vi "LEP_RV_InfoFile.vi"(0 "Path To Executable":path, 5 "Operation":u16(ring) items=["Read", "Write"], 7 "Item":string(combo), 9 "Data In":string, 11 "error in (no error)":errorcluster) -> (4 "Data Out":string, 15 "error out":errorcluster)   [LabVIEW 2011]
doc: "Loads project configuration information, creates the build folder, prepares the source files, builds, and links the embedded application."
uses:
  <vilib>/Utility/config.llb/Read Key (String).vi
  <vilib>/Utility/config.llb/Write Key (String).vi
  <vilib>/Utility/config.llb/NI_LVConfig.lvlib
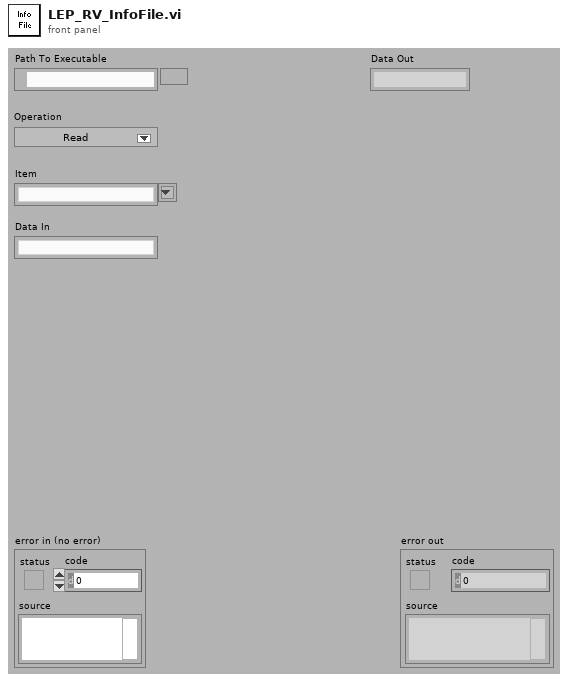
[diagram p1: front panel]
types:
  T1 = typedef "NI_LVConfig.lvlib/Config Data RefNum.ctl" = refnum<k1>
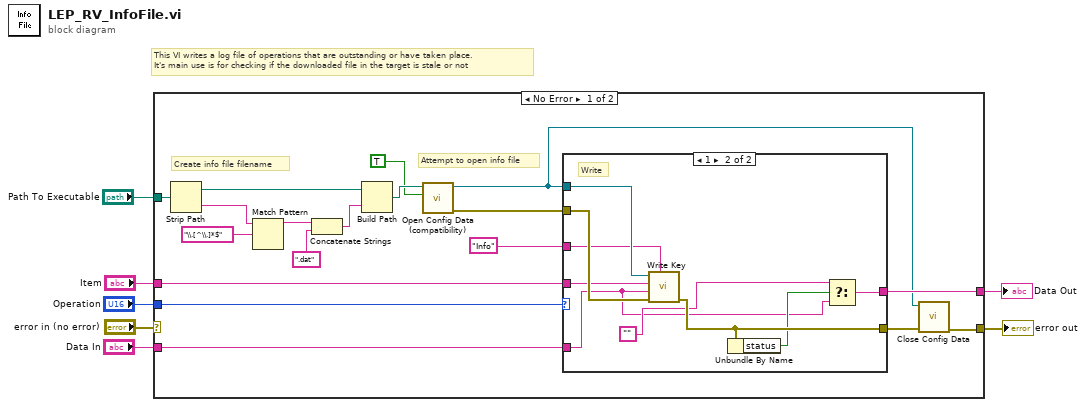
[diagram p0: block diagram]
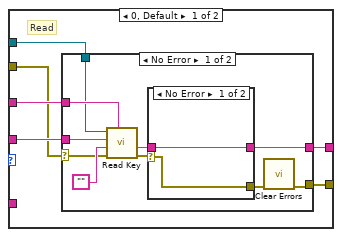
[diagram p2: hidden frame]
diagram:
  # "This VI writes a log file of operations that are outstanding or have taken place.\nIt's main use is for checking if the downloaded file in the target is stale or not"
  n1 = case shown="No Error" "error in (no error)" {
    selector: "error in (no error)" -> [_ w55]
    tunnel: [w10 w55] -> w5
    tunnel: "Path To Executable" -> [w25 _]
    tunnel: "Operation" -> [w16 _]
    tunnel: "Item" -> [w15 _]
    tunnel: [w12 _] -> w2
    tunnel: "Data In" -> [w8 _]
    frame No Error {
      # "Attempt to open info file"
      # "Create info file filename"
      n2 = Strip Path(path=w25) -> (stripped path=w23:path, name=w19:string)
      n3 = Match Pattern(string=w19, regular expression="\\.[^\\.]*$") -> (before substring=w21:string)  [unwired: 1 in, 3 out]
      n4 = Concatenate Strings(w21, ".dat" ("string")) -> (w24:string)
      n5 = Build Path(base path=w23, name or relative path=w24) -> (appended path=w18:path)
      n6 = call <vilib>:"Open Config Data (compatibility).vi"("create file if necessary (T)"=TRUE ("create file if necessary? (T)"), "configuration file path"=w18) -> ("error out"=w13:errorcluster, "refnum"=w9:T1)  [unwired: 7 in, 1 out]
      n7 = case shown="1" w16 {
        tunnel: w15 -> [w31 w48]
        tunnel: "Info" ("section") -> [w30 w52]
        tunnel: w13 -> [w26 w54]
        tunnel: w9 -> [w29 w53]
        tunnel: [w28 w49] -> w12
        tunnel: [w27 w51] -> w11
        tunnel: w8 -> [_ w46]
        frame 0, Default {
          # "Read"
          n8 = case shown="No Error" w26 {
            selector: w26 -> [w37 w45]
            tunnel: w31 -> [w41 _]
            tunnel: w30 -> [w40 _]
            tunnel: w29 -> [w39 _]
            tunnel: [w34 _] -> w28
            tunnel: [w36 w45] -> w27
            frame No Error {
              n9 = call-poly <vilib>:"Read Key.vi"("section"=w40, "error in (no error)"=w37, "default value"="", "key"=w41, "refnum"=w39) -> ("error out"=w35:errorcluster, "value"=w33:string)  [unwired: 3 in, 2 out]
              n10 = case shown="No Error" w35 {
                selector: w35 -> [w42 w44]
                tunnel: [w43 _] -> w34
                tunnel: w33 -> [w43 _]
                tunnel: [w42 w44] -> w32
                frame No Error {
                }
                frame Error {
                }
              }
              n11 = call <vilib>:"Clear Errors.vi"("error in (no error)"=w32) -> ("error out"=w36:errorcluster)  [unwired: 6 in]
            }
            frame Error {
            }
          }
        }
        frame 1 {
          # "Write"
          n12 = call-poly <vilib>:"Write Key.vi"("section"=w52, "error in (no error)"=w54, "value"=w46, "key"=w48, "refnum"=w53) -> ("error out"=w51:errorcluster)  [unwired: 4 in, 2 out]
          n13 = Unbundle By Name(w51) -> ("status"=w50:bool)
          n14 = Select(t="", s=w50, f=w46) -> (s? t:f=w49:string)
        }
      }
      n15 = call <vilib>:"Close Config Data.vi"("error in (no error)"=w11, "refnum"=w9) -> ("error out"=w10:errorcluster)  [unwired: 8 in, 1 out]
    }
    frame Error {
    }
  }
  "error out" <- w5
  "Data Out" <- w2
